vi "get_number_of_devices.vi"(11 "error in (no error)":errorcluster) -> (6 "num_of_devices (out)":i32, 15 "error out":errorcluster)   [LabVIEW 2012]
doc: "Retrieves the total number of attached devices. \n\nImplementss the USB Communication API function \"fnPerformaxComGetNumDevices\".\n\nProduced By:\n\nChristopher Lemieux\nKod Integrations, LLC\n4835 Marianne Drive\nMount Airy, MD 21771\nhttp://www.kodintegrations.com\nemail: clemieux@kodintegrations.com\nphone: (240) 687-1288"
uses:
  support/controls/errors_actions.ctl
  PerformaxCom.dll
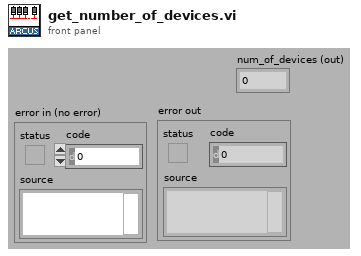
[diagram p1: front panel]
types:
  T1 = typedef "errors_actions.ctl" = enum16{"clearBuff", "closeRef", "noDeviceInfo", "noDevices", "openRef", "sendReceive", "setTimeouts", "unknown"}
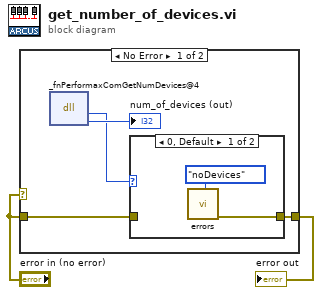
[diagram p0: block diagram]
diagram:
  n1 = case shown="No Error" "error in (no error)" {
    tunnel: [w4 w10] -> w2
    tunnel: "error in (no error)" -> [w3 w10]
    frame No Error {
      n2 = dll-call lib="PerformaxCom.dll" fn="_fnPerformaxComGetNumDevices@4"() -> (w5:i32, "numDevices"=→"num_of_devices (out)":i32)  [unwired: 4 in, 2 out]
      n3 = case shown="0, Default" w5 {
        tunnel: [w7 w9] -> w4
        tunnel: w3 -> [_ w9]
        frame 0, Default {
          n4 = call "errors.vi"("errors"=errors_actions."noDevices") -> ("error out"=w7:errorcluster)  [unwired: 14 in]
        }
        frame 1 {
        }
      }
    }
    frame Error {
    }
  }
  "error out" <- w2
